vi "Audio Device Playback Example (G-Audio).vi"() -> ()   [LabVIEW 2020]
doc: "Simple example of audio device playback of a file decoded with G-Audio."
uses:
  Controls/Audio Device Config.ctl
  Controls/Audio Device Format.ctl
  Controls/Audio Device Info.ctl
  Controls/Audio Device Type.ctl
  Audio Files/Polymorphic VIs/Get Audio File Info (Path).vi
  Audio Files/Polymorphic VIs/Open Audio File Read (Path).vi
  8289e2ef-86ba-4438-8a42-485f00fd8c95.vi
  9545a255-db38-479b-bcdc-619f4ee8d9ed.vi
  Private/Path To UTF-8 String.vi
  Audio Files/Private/Get Audio File Info (Core).vi
  Audio Files/Private/Open Audio File Read (Core).vi
  Private/Get Basic Audio File Info.vi
  Private/Result To Error.vi
  8289e2ef-86ba-4438-8a42-485f00fd8c95.vi/779dfdfd-1b42-4cf4-8001-66d3dd167625.vi
  8289e2ef-86ba-4438-8a42-485f00fd8c95.vi/55d550d4-9624-414e-aebd-6e02b5081896.vi
  9545a255-db38-479b-bcdc-619f4ee8d9ed.vi/4dfb5711-8d81-45a3-b3db-a84d40650863.vi
  9545a255-db38-479b-bcdc-619f4ee8d9ed.vi/c8869513-30c6-44f2-a2d3-73232fe63870.vi
  8289e2ef-86ba-4438-8a42-485f00fd8c95.vi/55d550d4-9624-414e-aebd-6e02b5081896.vi/4b7b629c-2e91-4160-9820-a26af8f6e677.vi
  9545a255-db38-479b-bcdc-619f4ee8d9ed.vi/4dfb5711-8d81-45a3-b3db-a84d40650863.vi/4b7b629c-2e91-4160-9820-a26af8f6e677.vi
  9545a255-db38-479b-bcdc-619f4ee8d9ed.vi/c8869513-30c6-44f2-a2d3-73232fe63870.vi/4b7b629c-2e91-4160-9820-a26af8f6e677.vi
  <vilib>/Utility/error.llb/Error Cluster From Error Code.vi
  <vilib>/Utility/Data Type/Get Numeric Information.vi
  G-Audio.lvlib
panel:
  out "Waveform":waveform(i16)[](graph)
  out "Now Playing:":string
  out "Duration":string
  out "Sample Length":u64
  out "Audio Info":T1
  out "error out":errorcluster
  in  "Stop":bool
  # "Instructions:\n1. Run the VI.\n2. Select an audio file to play.\n3. The VI will stop when the file has finished playing, or when the Stop button is pressed."
  # "G"
  # "-Audio"
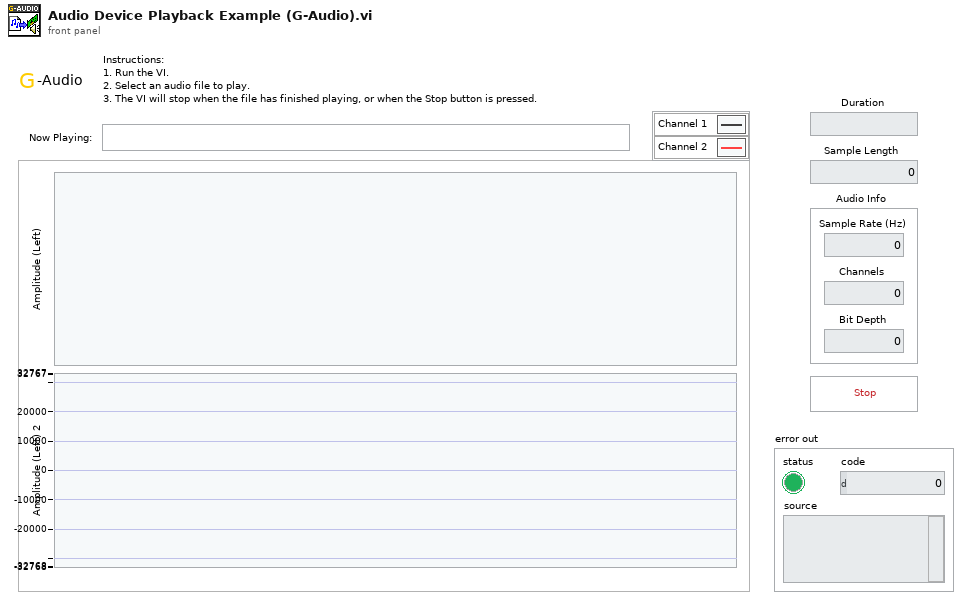
[diagram p1: front panel]
types:
  T1 = cluster{"Sample Rate (Hz)":u32, "Channels":u32, "Bit Depth":u32}
  T2 = typedef "G-Audio.lvlib/Audio Device Info.ctl" = cluster{"Name":string, "ID":u8[], "Device Type":T3}
  T3 = typedef "G-Audio.lvlib/Audio Device Type.ctl" = enum16{"(None)", "Playback", "Capture", "Duplex", "Loopback"}
  T4 = typedef "G-Audio.lvlib/Audio Device Config.ctl" = cluster{"Sample Rate (Hz)":u32, "Channels":u32, "Format":T5, "Exclusive Mode":bool}
  T5 = typedef "G-Audio.lvlib/Audio Device Format.ctl" = enum16{"Native", "U8", "I16", "I32", "SGL"}
  T6 = typedef "G-Audio.lvlib/Audio File Info.ctl" = cluster{"Sample Rate (Hz)":u32, "Channels":u32, "Bit Depth":u32}
  T7 = typedef "G-Audio.lvlib/Audio File Refnum.ctl" = refnum<file>
  T8 = typedef "G-Audio.lvlib/Audio Device Refnum.ctl" = refnum<file>
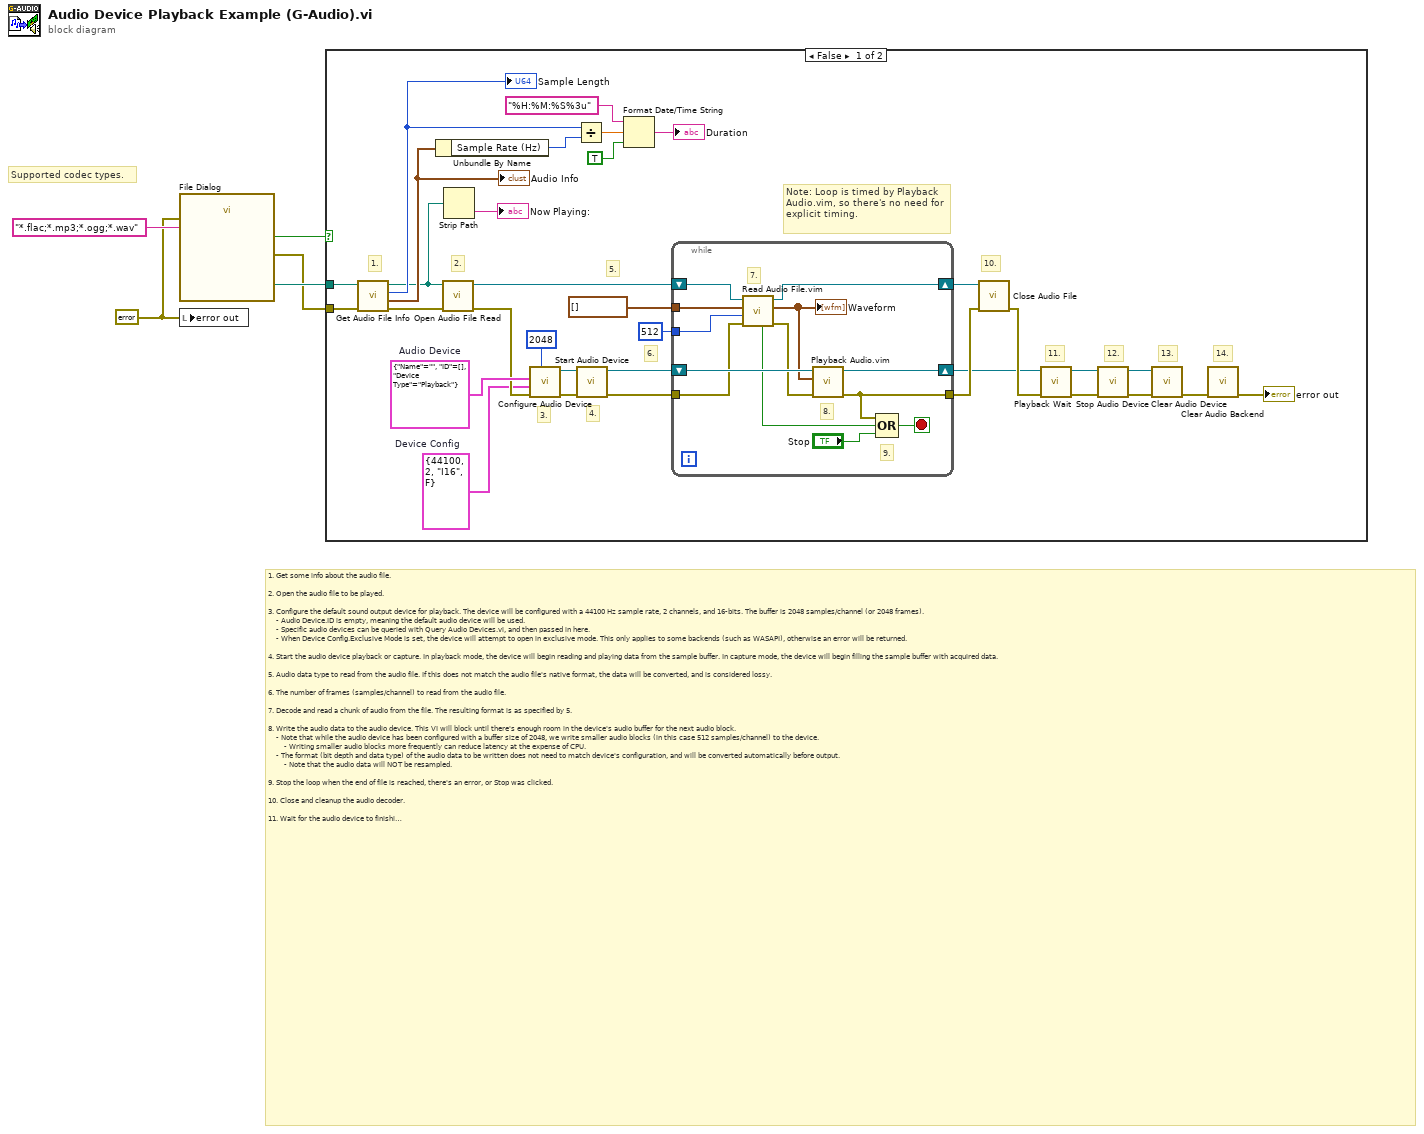
[diagram p0: block diagram]
diagram:
  w1 = errorcluster {"status"=FALSE, "code"=0, "source"=""} ("error out")
  # "1. Get some info about the audio file.\n\n2. Open the audio file to be played.\n\n3. Configure the default sound output device for playback. The device will be configured with a 44100 Hz sample rate, 2 channels, and 16-bits. The buffer is 2048 samples/channel (or 2048 frames).\n    - Audio Device.ID is empty, meaning the default audio device will be used.\n    - Specific audio devices can be queried with Query Audio Devices.vi, and then passed in here.\n    - When Device Config.Exclusive Mode is set, the device will attempt to open in exclusive mode. This only applies to some backends (such as WASAPI), otherwise an error will be returned.\n\n4. Start the audio device playback or capture. In playback mode, the device will begin reading and playing data from the sample buffer. In capture mode, the device will begin filling the sample buffer with acquired data.\n\n5. Audio data type to read from the audio file. If this does not match the audio file's native format, the data will be converted, and is considered lossy.\n\n6. The number of frames (samples/channel) to read from the audio file.\n\n7. Decode and read a chunk of audio from the file. The resulting format is as specified by 5.\n\n8. Write the audio data to the audio device. This VI will block until there's enough room in the device's audio buffer for the next audio block.\n    - Note that while the audio device has been configured with a buffer size of 2048, we write smaller audio blocks (in this case 512 samples/channel) to the device.\n        - Writing smaller audio blocks more frequently can reduce latency at the expense of CPU.\n    - The format (bit depth and data type) of the audio data to be written does not need to match device's configuration, and will be converted automatically before output.\n        - Note that the audio data will NOT be resampled.\n\n9. Stop the loop when the end of file is reached, there's an error, or Stop was clicked.\n\n10. Close and cleanup the audio decoder.\n\n11. Wait for the audio device to finishing playing the content of the audio buffer.\n\n12. Stop the audio device.\n    - This function isn't strictly required, as Clear Audio Device.vi will implicitly stop the audio device. It's shown here to demonstrate the available API.\n    - Stopping the device does not clear or reset the audio buffer. If it is started again with Start Audio Device.vi, playback will resume.\n\n13. Clear the device and audio buffer. The device will become invalid.\n\n14. Clear the audio backend.\n    - Clearing the backend will forcibly stop all audio devices configured on that backend. It's only necessary to clear the backend if you wish to switch to another backend."
  # "Supported codec types."
  n1 = call "File Dialog"("error in"=w1, "pattern (all files)"="*.flac;*.mp3;*.ogg;*.wav") -> ("selected path"=w4:path, "cancelled"=w3:bool, "error out"=w2:errorcluster)  [unwired: 10 in, 1 out]
  n2 = local write "error out"(w1) -> ()
  n3 = case shown="False" w3 {
    tunnel: w4 -> [w8 _]
    tunnel: w2 -> [w38 _]
    frame False {
      w13 = T2 {"Name"="", "ID"=[], "Device Type"=enum."Playback"}  # Audio Device
      w11 = T4 {"Sample Rate (Hz)"=44100, "Channels"=2, "Format"=enum."I16", "Exclusive Mode"=FALSE}  # Device Config
      # "14."
      # "13."
      # "12."
      # "11."
      # "10."
      # "6."
      # "4."
      # "Note: Loop is timed by Playback Audio.vim, so there's no need for explicit timing."
      # "5."
      # "3."
      # "2."
      # "1."
      n4 = call-poly "Get Audio File Info.vi"("error in (no error)"=w38, "Path In"=w8) -> ("error out"=w37:errorcluster, "Audio File Info"=w25:T6, "PCM Frame Length"=w26:u64, "Path Out"=w7:path)  [unwired: 5 in, 1 out]
      "Audio Info" <- w25
      "Sample Length" <- w26
      n5 = Unbundle By Name(w25) -> ("Sample Rate (Hz)"=w24:u32)
      n6 = call-poly "Open Audio File Read.vi"("error in (no error)"=w37, "Path"=w7) -> ("error out"=w12:errorcluster, "Audio File Refnum"=w28:T7)  [unwired: 8 in]
      n7 = Strip Path(path=w7) -> (name=→"Now Playing:":string)  [unwired: 1 out]
      n8 = call "Configure Audio Device.vi"("Buffer Size (4096)"=2048 ("number of samples/ch"), "error in (no error)"=w12, "Device Config"=w11, "Audio Device"=w13) -> ("error out"=w19:errorcluster, "Audio Device Refnum"=w18:T8)  [unwired: 6 in]
      n9 = Divide(x=w26, y=w24) -> (x/y=w23:dbl)
      n10 = call "Start Audio Device.vi"("error in (no error)"=w19, "Audio Device Refnum In"=w18) -> ("error out"=w30:errorcluster, "Audio Device Refnum Out"=w31:T8)  [unwired: 8 in]
      n11 = Format Date/Time String(time format string (%c)="%H:%M:%S%3u", seconds (now)=w23, UTC format=TRUE) -> (date/time string=→"Duration":string)
      n12 = while {
        shift-right: [w49] -> w36
        shift-left: w28 -> [w51]
        shift-right: [w48] -> w15
        shift-left: w31 -> [w50]
        tunnel: w30 -> [w47]
        tunnel: [w42] -> w34
        tunnel: u64 512 ("number of samples/ch") -> [w41]
        tunnel: waveform(i16)[] [] -> [w40]
        stop <- w44 stop-if-true
        # "9."
        # "8."
        # "7."
        n13 = call "Read Audio File.vim"("error in (no error)"=w47, "Frames To Read"=w41, "Data Format"=w40, "Audio File Refnum In"=w51) -> ("error out"=w46:errorcluster, "Audio Data"=w39:waveform(i16)[], "Audio File Refnum Out"=w49:T7, "End of File?"=w45:bool)  [unwired: 3 in, 1 out]
        "Waveform" <- w39
        n14 = call "Playback Audio.vim"("error in (no error)"=w46, "Audio Data"=w39, "Audio Device Refnum In"=w50) -> ("error out"=w42:errorcluster, "Audio Device Refnum Out"=w48:T8)  [unwired: 7 in]
        n15 = Compound Arithmetic op=OR(w42, w45, "Stop") -> (w44:bool)
      }
      n16 = call "Close Audio File.vi"("error in (no error)"=w34, "Audio File Refnum In"=w36) -> ("error out"=w33:errorcluster)  [unwired: 9 in]
      n17 = call "Playback Wait.vi"("error in (no error)"=w33, "Audio Device Refnum In"=w15) -> ("error out"=w16:errorcluster, "Audio Device Refnum Out"=w14:T8)  [unwired: 8 in]
      n18 = call "Stop Audio Device.vi"("error in (no error)"=w16, "Audio Device Refnum In"=w14) -> ("error out"=w32:errorcluster, "Audio Device Refnum Out"=w35:T8)  [unwired: 8 in]
      n19 = call "Clear Audio Device.vi"("error in (no error)"=w32, "Audio Device Refnum In"=w35) -> ("error out"=w29:errorcluster)  [unwired: 9 in]
      n20 = call "Clear Audio Backend.vi"("error in (no error)"=w29) -> ("error out"=→"error out":errorcluster)  [unwired: 10 in]
    }
    frame True {
    }
  }
